vi "Update Channel Properties.vi"(8 "error in (no error)":errorcluster, 10 "Signal In":T1, 11 "nodeID In":u64) -> (0 "error out":errorcluster)   [LabVIEW 2025]
uses:
  <vilib>/Vehicle Communication Toolkit/TypDefs/RBS Signal.ctl
  <vilib>/NI/NI VeriStand Advanced SysDef API/_SubVIs/SysDef.Property.Set.U32.vi
  <vilib>/NI/NI VeriStand Advanced SysDef API/_SubVIs/SysDef.Property.Set.DBL.vi
  <vilib>/NI/NI VeriStand Advanced SysDef API/SysDef API/Advanced System Definition.lvlib
  <vilib>/Vehicle Communication Toolkit/Vehicle Communication Toolkit.lvlib
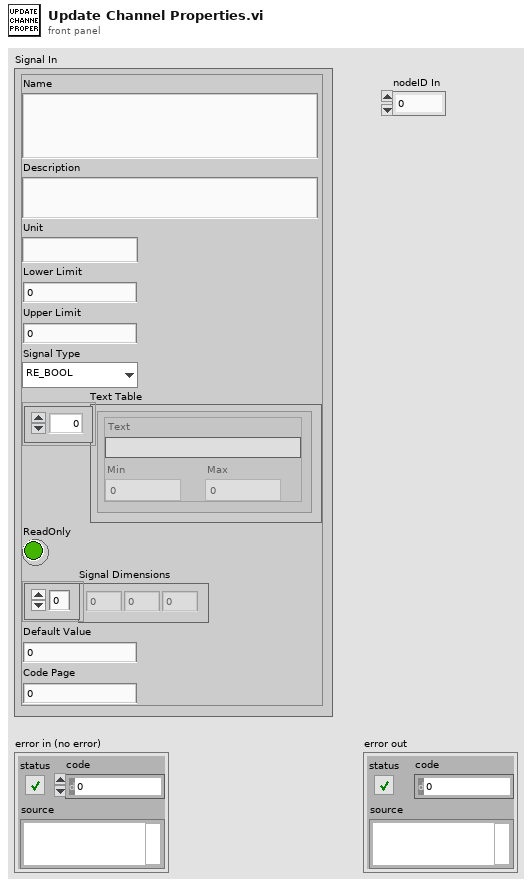
[diagram p1: front panel]
types:
  T1 = typedef "Vehicle Communication Toolkit.lvlib/RBS Signal.ctl" = cluster{"Name":string, "Description":string, "Unit":string, "Lower Limit":dbl, "Upper Limit":dbl, "Signal Type":enum32{"RE_BOOL", "RE_UINT8", "RE_INT8", "RE_UINT16", "RE_INT16", "RE_UINT32", "RE_INT32", "RE_UINT64", "RE_INT64", "RE_FLOAT32", "RE_FLOAT64", "RE_TEXT"}, "Text Table":cluster{"Text":string, "Min":dbl, "Max":dbl}[], "ReadOnly":bool, "Signal Dimensions":u32[], "Default Value":dbl, "Code Page":u32}
  T2 = enum32{"RE_BOOL", "RE_UINT8", "RE_INT8", "RE_UINT16", "RE_INT16", "RE_UINT32", "RE_INT32", "RE_UINT64", "RE_INT64", "RE_FLOAT32", "RE_FLOAT64", "RE_TEXT"}
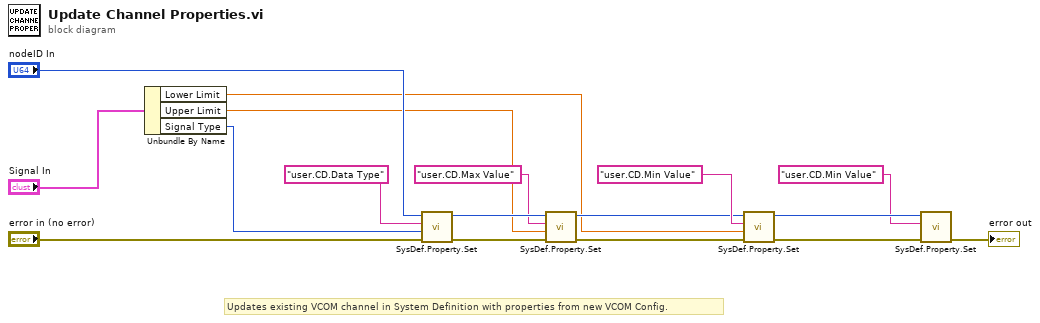
[diagram p0: block diagram]
diagram:
  # "Updates existing VCOM channel in System Definition with properties from new VCOM Config."
  n1 = Unbundle By Name("Signal In") -> ("Lower Limit"=w1:dbl, "Upper Limit"=w2:dbl, "Signal Type"=w14:T2)
  n2 = call-poly <vilib>:"SysDef.Property.Set.vi"("error in (no error)"="error in (no error)", "Value"=w14, "Property Name"="user.CD.Data Type", "nodeID"="nodeID In") -> ("error out"=w11:errorcluster, "nodeID out"=w12:u64)  [unwired: 6 in]
  n3 = call-poly <vilib>:"SysDef.Property.Set.vi"("error in (no error)"=w11, "Value"=w2, "Property Name"="user.CD.Max Value", "nodeID"=w12) -> ("error out"=w9:errorcluster, "nodeID out"=w5:u64)  [unwired: 6 in]
  n4 = call-poly <vilib>:"SysDef.Property.Set.vi"("error in (no error)"=w9, "Value"=w1, "Property Name"="user.CD.Min Value", "nodeID"=w5) -> ("error out"=w10:errorcluster, "nodeID out"=w4:u64)  [unwired: 6 in]
  n5 = call-poly <vilib>:"SysDef.Property.Set.vi"("error in (no error)"=w10, "Property Name"="user.CD.Min Value", "nodeID"=w4) -> ("error out"=→"error out":errorcluster)  [unwired: 7 in, 1 out]
